vi "Sample Changer 4032 tester.vi"() -> ()   [LabVIEW 2016]
uses:
  Tester-states.ctl
  <vilib>/Utility/file.llb/Write Delimited Spreadsheet (string).vi
  <vilib>/Utility/file.llb/Write Delimited Spreadsheet (I64).vi
  <vilib>/Analysis/NI_AALBase.lvlib
panel:
  in  "file path (dialog if empty)":path
  out "Target Attempts":i32(graph)
  out "Rotation time vs Target Attempts":cluster{i32, i32}[](graph)
  out "Encoder distance":i32
  out "Start Position":i32
  out "output array":cluster{u32, i32}[](array[cluster])
  out "Time vs Distance cluster":cluster{u32, i32}
  out "Rotation time vs Encoder distance":cluster{i32, i32}[](graph)
  in  "Rotation Timeout (ms)":dbl=30000.0
  out "Rotation Duration":u32(graph)
  out "Rotation Duration Histogram":T1(graph)
  out "End Time":timestamp
  out "Start Time":timestamp
  out "Error Histogram":T1(graph)
  out "Success rate":dbl
  out "Sample Number":cluster{"UInt8":u8, "UInt8":u8}(graph)
  in  "Rotate minimum time (ms)":u32=5000
  out "Position error (encoder steps)":i32(graph)
  out "Encoder data":cluster{"Int32":i32, "Int32":i32}(graph)={"Int32"=515, "Int32"=0}
  out "Encoder Destination":i32
  out "Encoder Position":i32
  out "Current Sample":u8
  out "Loop Counter":i32
  in  "Encoder Radius":dbl=2.0
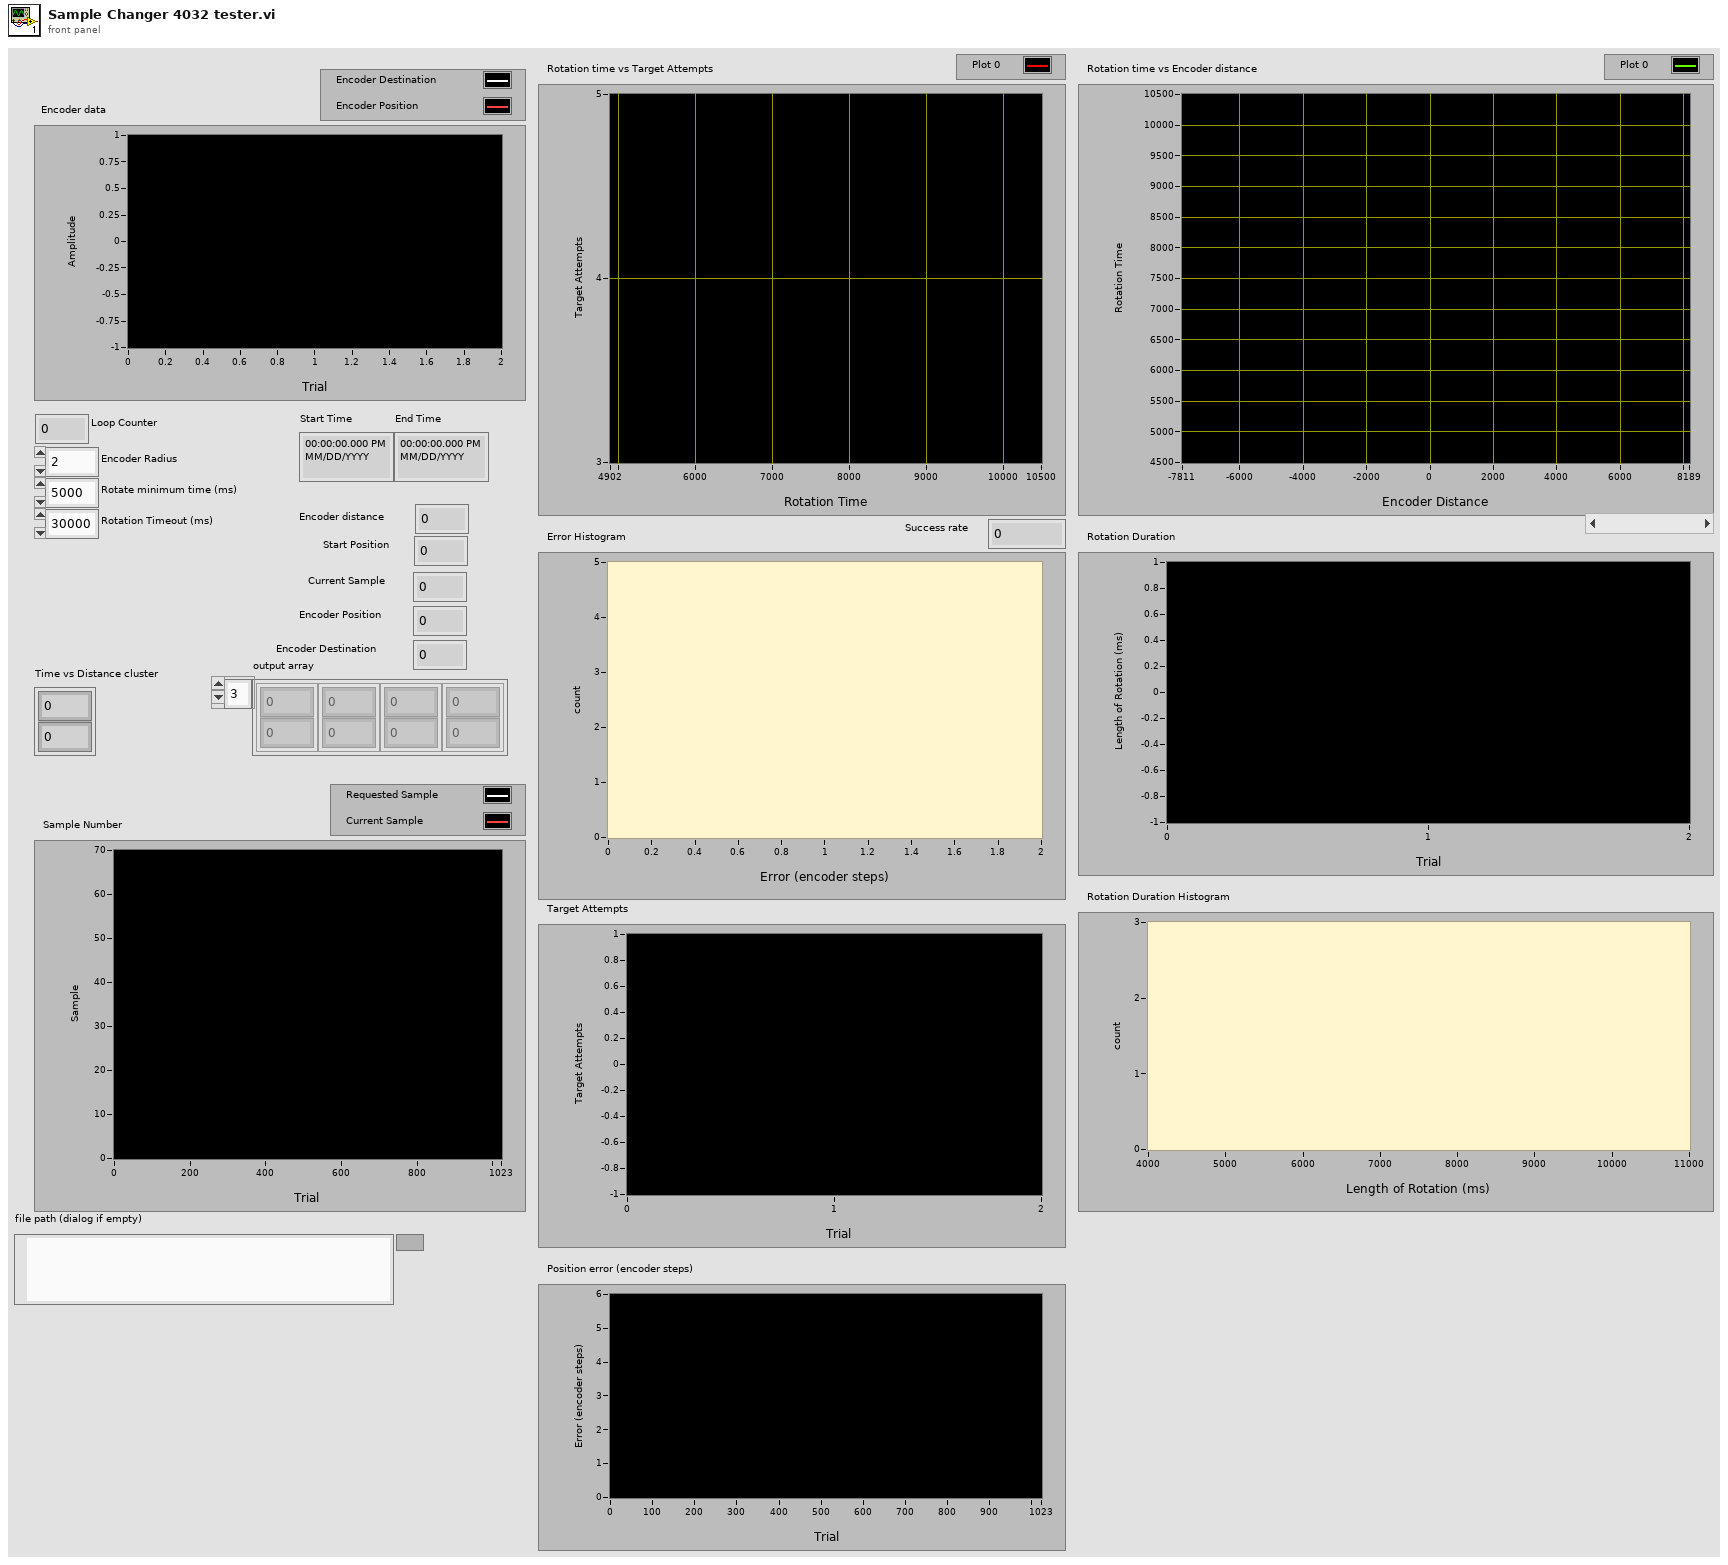
[diagram p1: front panel]
types:
  T1 = cluster{"X Values":dbl[], "Histogram: h(x)":i32[]}
  T2 = typedef "Tester-states.ctl" = enum16{"wait", "start trial", "get trial data", "test complete"}
  T3 = cluster{i32, i32, "Int32":i32, i32, i32, i32, i32}
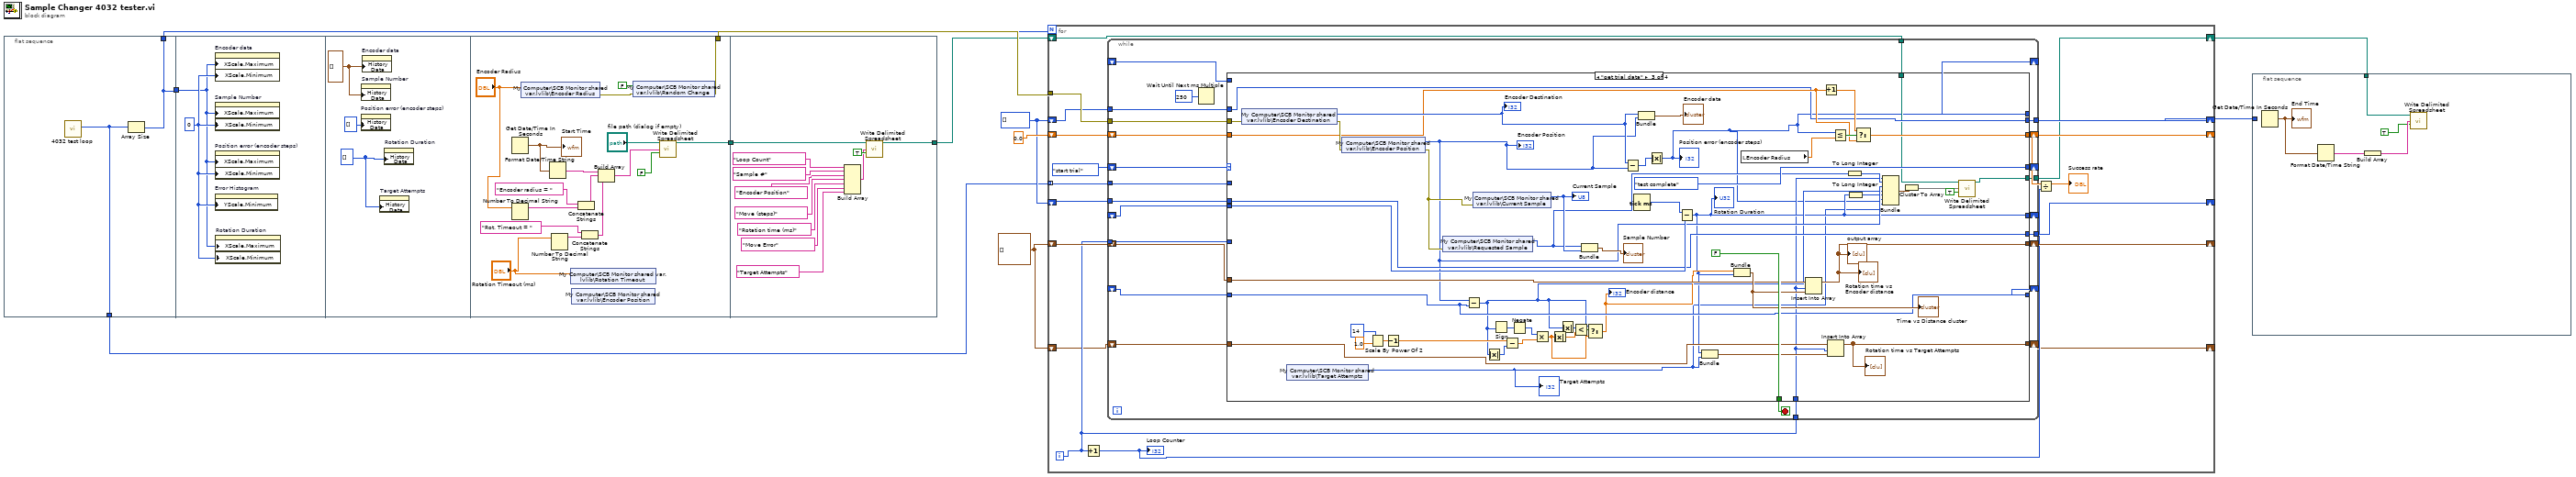
[diagram p0: block diagram]
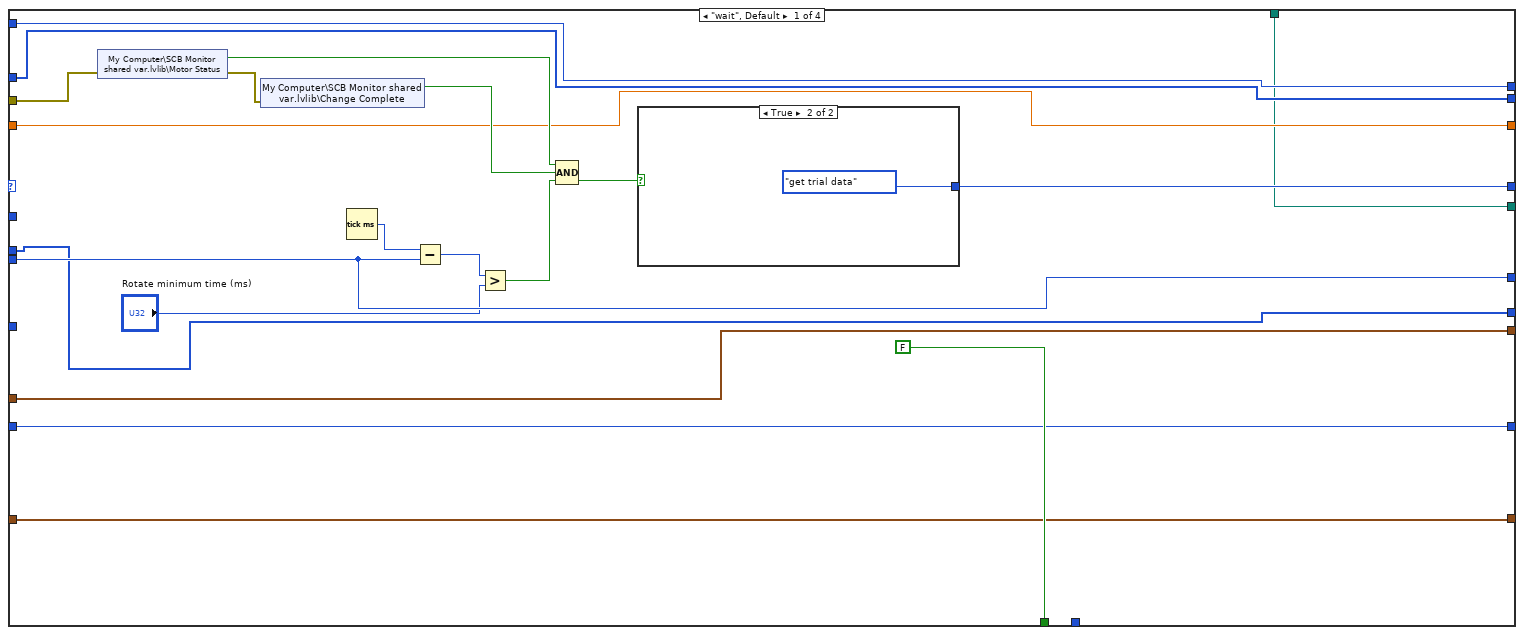
[diagram p2: hidden frame]
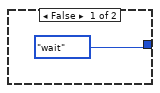
[diagram p3: hidden frame]
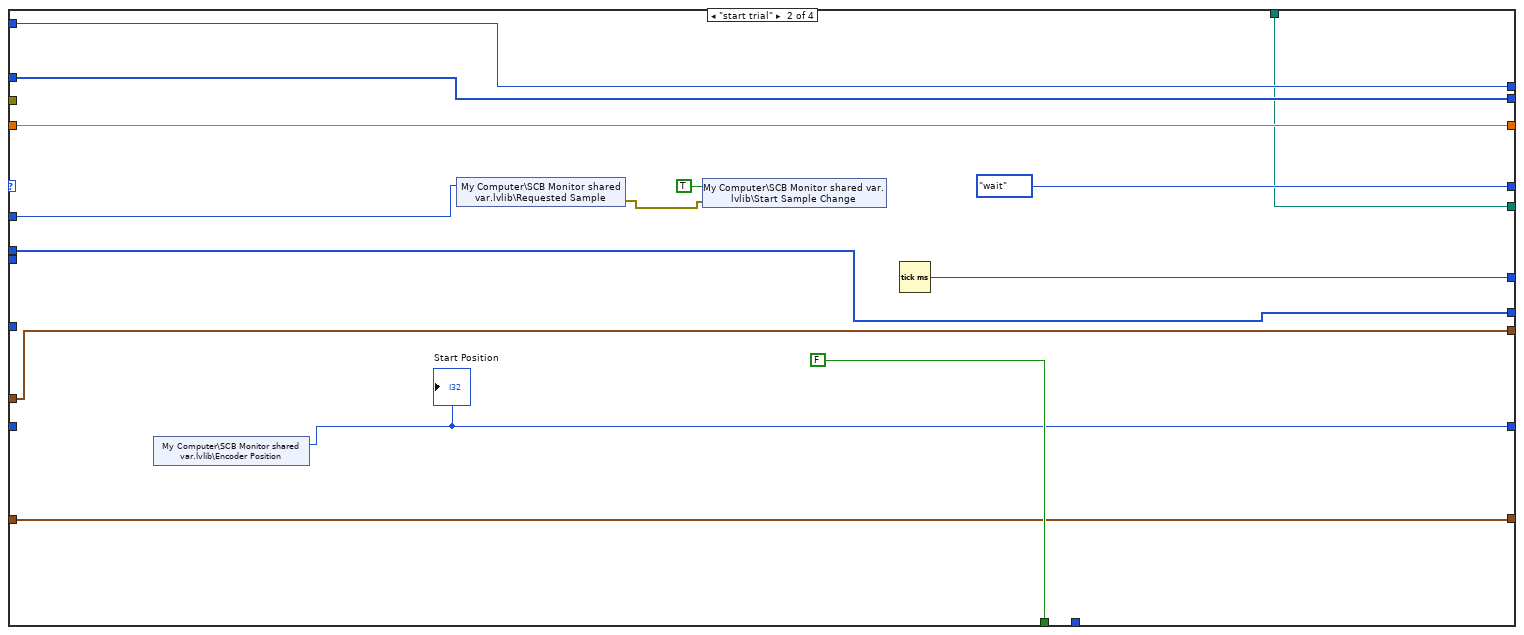
[diagram p4: hidden frame]
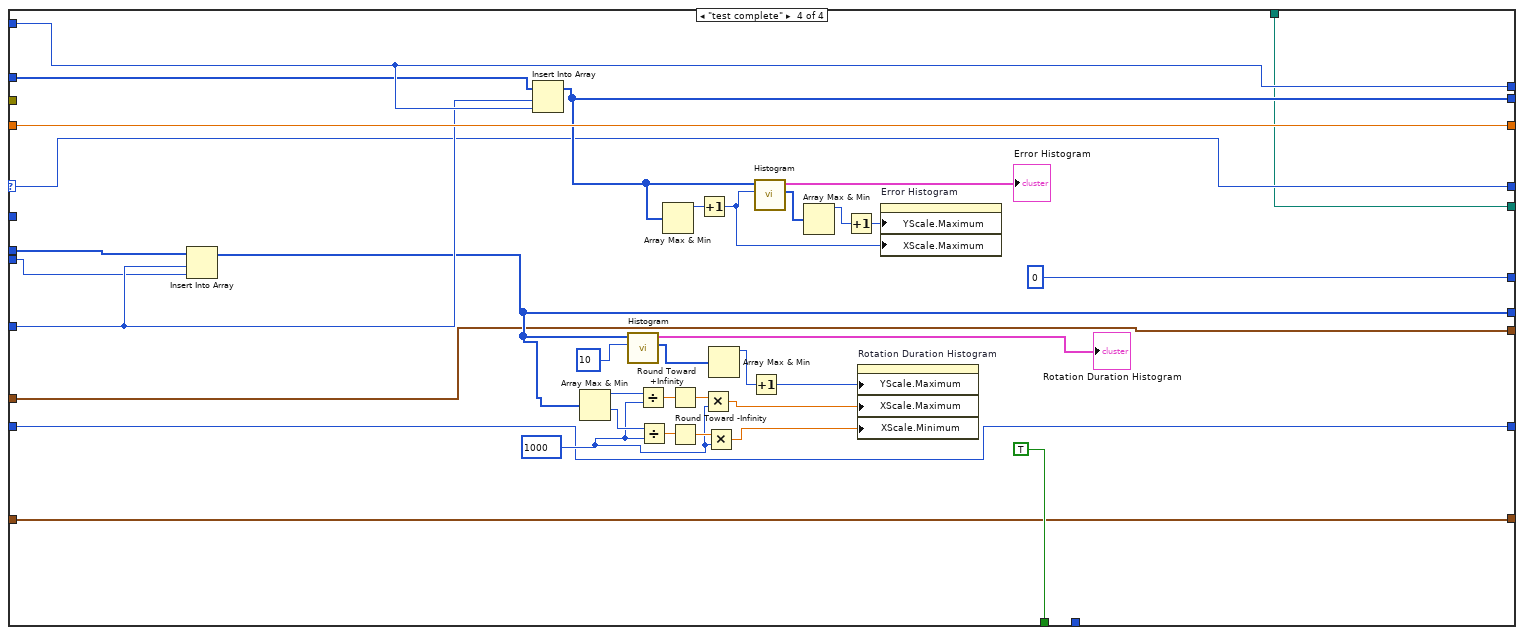
[diagram p5: hidden frame]
diagram:
  w4 = cluster{i32, i32}[] []
  w8 = i32[] []
  n1 = flat-sequence {
    tunnel: [w12] -> w7
    tunnel: [w13] -> w6
    tunnel: [w12] -> w5
    tunnel: w7 -> [w14]
    tunnel: [w33] -> w11
    tunnel: [w31] -> w1
    tunnel: [w45] -> w3
    tunnel: w1 -> [w46]
    frame #0 {
      n2 = call "4032 test loop.vi"() -> ("Array"=w13:i32[])  [unwired: 10 in]
      n3 = Array Size(array=w13) -> (size(s)=w12:i32)
    }
    frame #1 {
      w15 = 0 ("Trials 2")
      n4 = property on="Encoder data" class="WFChart (strict)"("XScale.Maximum"=w14, "XScale.Minimum"=w15) -> ()  [unwired: 2 in, 2 out]
      n5 = property on="Sample Number" class="WFChart (strict)"("XScale.Maximum"=w14, "XScale.Minimum"=w15) -> ()  [unwired: 2 in, 2 out]
      n6 = property on="Position error (encoder steps)" class="WFChart (strict)"("XScale.Maximum"=w14, "XScale.Minimum"=w15) -> ()  [unwired: 2 in, 2 out]
      n7 = property on="Error Histogram" class="XYGraph (strict)"("YScale.Minimum"=w15) -> ()  [unwired: 2 in, 2 out]
      n8 = property on="Rotation Duration" class="WFChart (strict)"("XScale.Maximum"=w14, "XScale.Minimum"=w15) -> ()  [unwired: 2 in, 2 out]
    }
    frame #2 {
      w16 = i32[] [] ("History Data")
      w17 = cluster{"Int32":i32, "Int32":i32}[] [] ("History Data")
      n9 = property on="Position error (encoder steps)" class="WFChart (strict)"("History Data"=i32[] []) -> ()  [unwired: 2 in, 2 out]
      n10 = property on="Sample Number" class="WFChart (strict)"("History Data"=w17) -> ()  [unwired: 2 in, 2 out]
      n11 = property on="Encoder data" class="WFChart (strict)"("History Data"=w17) -> ()  [unwired: 2 in, 2 out]
      n12 = property on="Target Attempts" class="WFChart (strict)"("History Data"=w16) -> ()  [unwired: 2 in, 2 out]
      n13 = property on="Rotation Duration" class="WFChart (strict)"("History Data"=w16) -> ()  [unwired: 2 in, 2 out]
    }
    frame #3 {
      n14 = Get Date/Time In Seconds() -> (seconds since 1Jan1904=w30:timestamp)
      "Start Time" <- w30
      n15 = Number To Decimal String(number="Encoder Radius") -> (decimal integer string=w24:string)  [unwired: 1 in]
      n16 = shared-variable "My Computer\\SCB Monitor shared var.lvlib\\Encoder Radius"("Encoder Radius") -> (error out=w35:errorcluster)  [unwired: 1 in]
      n17 = Format Date/Time String(seconds (now)=w30) -> (date/time string=w29:string)  [unwired: 2 in]
      n18 = Number To Decimal String(number="Rotation Timeout (ms)") -> (decimal integer string=w21:string)  [unwired: 1 in]
      n19 = shared-variable "My Computer\\SCB Monitor shared var.lvlib\\Rotation Timeout"("Rotation Timeout (ms)") -> ()  [unwired: 1 in, 1 out]
      n20 = shared-variable "My Computer\\SCB Monitor shared var.lvlib\\Encoder Position"() -> ()  [unwired: 1 in, 2 out]
      n21 = Concatenate Strings("Encoder radius = ", w24) -> (w23:string)
      n22 = Concatenate Strings("Rot. Timeout = ", w21) -> (w19:string)
      n23 = Build Array(w29, w23, w19) -> (w28:string[])
      n24 = shared-variable "My Computer\\SCB Monitor shared var.lvlib\\Random Change"(FALSE ("Random Change"), error in=w35) -> (error out=w33:errorcluster)
      n25 = call-poly <vilib>:"Write Delimited Spreadsheet.vi"("file path (dialog if empty)"="file path (dialog if empty)", "1D data"=w28, "append to file? (new file:F)"=FALSE) -> ("new file path (Not A Path if cancelled)"=w31:path)  [unwired: 11 in, 1 out]
    }
    frame #4 {
      n26 = Build Array("Loop Count", "Sample #", "Encoder Position", "Move (steps)", "Rotation time (ms)", "Move Error", "Target Attempts" ("element")) -> (w43:string[])
      n27 = call-poly <vilib>:"Write Delimited Spreadsheet.vi"("file path (dialog if empty)"=w46, "1D data"=w43, "append to file? (new file:F)"=TRUE) -> ("new file path (Not A Path if cancelled)"=w45:path)  [unwired: 11 in, 1 out]
    }
  }
  n28 = for {
    N: w5 -> [_]
    tunnel: w11 -> [w63]
    shift-right: [w60] -> _
    shift-left: 0.0 -> [w62]
    shift-right: [w59] -> w9
    shift-left: w8 -> [w58]
    shift-right: [w56] -> _
    shift-left: w8 -> [w57]
    shift-right: [w55] -> _
    shift-left: w4 -> [w54]
    tunnel: w6 -> [w52] mode=indexing
    shift-right: [w49] -> _
    shift-left: w4 -> [w51]
    shift-right: [w47] -> w2
    shift-left: w3 -> [w48]
    i -> [w53]
    n29 = Increment(x=w53) -> (x+1=w50:i32)
    "Loop Counter" <- w50
    n30 = while {
      shift-right: [w88] -> _
      shift-left: Tester-states."start trial" -> [w87]
      tunnel: w63 -> [w86]
      shift-right: [w85] -> _
      shift-left: _ -> [w84]
      shift-right: [w82] -> _
      shift-left: _ -> [w83]
      shift-right: [w81] -> w60
      shift-left: w62 -> [w80]
      tunnel: w53 -> [w79]
      tunnel: [w78] -> w59
      tunnel: w58 -> [w77]
      tunnel: w57 -> [w76]
      tunnel: [w75] -> w56
      tunnel: w53 -> [w71]
      shift-right: [w73] -> w55
      shift-left: w54 -> [w72]
      tunnel: w52 -> [w70]
      shift-right: [w74] -> _
      shift-left: _ -> [w69]
      shift-right: [w68] -> w49
      shift-left: w51 -> [w67]
      tunnel: w48 -> [w66]
      tunnel: [w65] -> w47
      stop <- w90 stop-if-true
      n31 = Wait Until Next ms Multiple(millisecond multiple=u32 250) -> ()  [unwired: 1 out]
      n32 = case shown="\"get trial data\"" w87 {
        selector: w87 -> [_ _ _ w199]
        tunnel: [FALSE FALSE FALSE TRUE] -> w90
        tunnel: [w109 Tester-states."wait" Tester-states."test complete" w199] -> w88
        tunnel: w86 -> [w101 _ w175 _]
        tunnel: [w103 w122 w137 u32 0 ("millisecond timer value")] -> w85
        tunnel: w84 -> [w103 _ w162 w201]
        tunnel: w83 -> [w98 w121 _ w211]
        tunnel: [w98 w121 w127 w211] -> w82
        tunnel: [w97 w120 w167 w212] -> w81
        tunnel: w80 -> [w97 w120 w166 w212]
        tunnel: w79 -> [_ _ _ w202]
        tunnel: [w96 w119 w164 w203] -> w78
        tunnel: w77 -> [w96 w119 w164 w210]
        tunnel: w76 -> [w95 w118 w161 w200]
        tunnel: [w95 w118 w161 w193] -> w75
        tunnel: [w93 w115 w157 w182] -> w74
        tunnel: w69 -> [w93 _ w157 w182]
        tunnel: [w94 w117 w158 w183] -> w73
        tunnel: w72 -> [w94 w117 w159 w183]
        tunnel: w71 -> [_ _ w131 _]
        tunnel: w70 -> [_ w116 _ _]
        tunnel: [w92 w114 w141 w181] -> w68
        tunnel: w67 -> [w92 w114 w142 w181]
        tunnel: w66 -> [w91 w113 w132 w180]
        tunnel: [w91 w113 w130 w180] -> w65
        frame "wait", Default {
          n33 = shared-variable "My Computer\\SCB Monitor shared var.lvlib\\Motor Status"(error in=w101) -> (w102:bool, error out=w100:errorcluster)
          n34 = shared-variable "My Computer\\SCB Monitor shared var.lvlib\\Change Complete"(error in=w100) -> (w106:bool)  [unwired: 1 out]
          n35 = Tick Count (ms)() -> (millisecond timer value=w108:u32)
          n36 = Subtract(x=w108, y=w103) -> (x-y=w105:u32)
          n37 = Greater?(x=w105, y="Rotate minimum time (ms)") -> (0:w104:bool)
          n38 = Compound Arithmetic op=AND(w102, w106, w104) -> (w107:bool)
          n39 = case shown="True" w107 {
            tunnel: [Tester-states."wait" Tester-states."get trial data"] -> w109
            frame False {
            }
            frame True {
            }
          }
        }
        frame "start trial" {
          n40 = shared-variable "My Computer\\SCB Monitor shared var.lvlib\\Encoder Position"() -> (w115:i32)  [unwired: 1 in, 1 out]
          "Start Position" <- w115
          n41 = shared-variable "My Computer\\SCB Monitor shared var.lvlib\\Requested Sample"(w116) -> (error out=w123:errorcluster)  [unwired: 1 in]
          n42 = shared-variable "My Computer\\SCB Monitor shared var.lvlib\\Start Sample Change"(TRUE ("Start Sample Change"), error in=w123) -> ()  [unwired: 1 out]
          n43 = Tick Count (ms)() -> (millisecond timer value=w122:u32)
        }
        frame "get trial data" {
          n44 = shared-variable "My Computer\\SCB Monitor shared var.lvlib\\Encoder Destination"(error in=w175) -> (w173:i32, error out=w174:errorcluster)
          "Encoder Destination" <- w173
          n45 = shared-variable "My Computer\\SCB Monitor shared var.lvlib\\Target Attempts"() -> (w128:i32)  [unwired: 1 in, 1 out]
          "Target Attempts" <- w128
          n46 = shared-variable "My Computer\\SCB Monitor shared var.lvlib\\Encoder Position"(error in=w174) -> (w139:i32, error out=w172:errorcluster)
          "Encoder Position" <- w139
          n47 = Scale By Power Of 2(n=i16 14, x=1.0) -> (x*2^n=w154:dbl)
          n48 = Decrement(x=w154) -> (x-1=w153:dbl)
          n49 = shared-variable "My Computer\\SCB Monitor shared var.lvlib\\Requested Sample"(error in=w172) -> (w140:u8)  [unwired: 1 out]
          n50 = Subtract(x=w139, y=w157) -> (x-y=w138:i32)
          n51 = shared-variable "My Computer\\SCB Monitor shared var.lvlib\\Current Sample"(error in=w172) -> (w170:u8)  [unwired: 1 out]
          "Current Sample" <- w170
          n52 = Absolute Value(x=w138) -> (abs(x)=w152:i32)
          n53 = Sign(1:w138) -> (0:w150:i32)
          n54 = Subtract(x=w153, y=w152) -> (x-y=w151:dbl)
          n55 = Negate(x=w150) -> (-x=w149:i32)
          n56 = Multiply(x=w149, y=w151) -> (x*y=w145:dbl)
          n57 = Absolute Value(x=w145) -> (abs(x)=w148:dbl)
          n58 = Absolute Value(x=w138) -> (abs(x)=w147:i32)
          n59 = Less?(x=w147, y=w148) -> (x < y?=w146:bool)
          n60 = Bundle("UInt8"=w140, "UInt8"=w170) -> (→"Sample Number":cluster{"UInt8":u8, "UInt8":u8})  [unwired: 1 in]
          n61 = Select(t=w138, s=w146, f=w145) -> (s? t:f=w144:dbl)
          "Encoder distance" <- w144
          n62 = Subtract(x=w173, y=w139) -> (x-y=w177:i32)
          n63 = Tick Count (ms)() -> (millisecond timer value=w163:u32)
          n64 = Bundle("Int32"=w173, "Int32"=w139) -> (→"Encoder data":cluster{"Int32":i32, "Int32":i32})  [unwired: 1 in]
          n65 = Absolute Value(x=w177) -> (abs(x)=w127:i32)
          "Position error (encoder steps)" <- w127
          n66 = Subtract(x=w163, y=w162) -> (x-y=w137:u32)
          "Rotation Duration" <- w137
          n67 = Bundle(w137, w128) -> (w143:cluster{u32, i32})  [unwired: 1 in]
          n68 = Bundle(w144, w137) -> (w160:cluster{dbl, u32})  [unwired: 1 in]
          "Time vs Distance cluster" <- w160
          n69 = local read "Encoder Radius"() -> (w169:dbl)
          n70 = Insert Into Array(array=w159, index=w131, new element=w160) -> (w158:cluster{i32, i32}[])
          "Rotation time vs Encoder distance" <- w158
          "output array" <- w158
          n71 = Increment(x=w166) -> (x+1=w165:dbl)
          n72 = Insert Into Array(array=w142, index=w131, new element=w143) -> (w141:cluster{i32, i32}[])
          "Rotation time vs Target Attempts" <- w141
          n73 = Less Or Equal?(x=w127, y=w169) -> (x <= y?=w168:bool)
          n74 = To Long Integer(number=w140) -> (32bit integer=w136:i32)
          n75 = To Long Integer(number=w137) -> (32bit integer=w135:i32)
          n76 = Select(t=w165, s=w168, f=w166) -> (s? t:f=w167:dbl)
          n77 = Bundle(w131, w136, "Int32"=w139, w138, w135, w127, w128) -> (w134:T3)  [unwired: 1 in]
          n78 = Cluster To Array(cluster=w134) -> (array=w133:i32[])
          n79 = call-poly <vilib>:"Write Delimited Spreadsheet.vi"("file path (dialog if empty)"=w132, "1D data"=w133, "append to file? (new file:F)"=TRUE) -> ("new file path (Not A Path if cancelled)"=w130:path)  [unwired: 11 in, 1 out]
        }
        frame "test complete" {
          w186 = 1000 ("y")
          n80 = Insert Into Array(array=w200, index=w202, new element=w201) -> (w193:i32[])
          n81 = Insert Into Array(array=w210, index=w202, new element=w211) -> (w203:i32[])
          n82 = Array Max & Min(array=w193) -> (max value=w192:i32, min value=w191:i32)  [unwired: 2 out]
          n83 = call <vilib>:"Histogram.vi"("intervals"=10, "X"=w193) -> ("Histogram: h(x)"=w195:i32[], "Histogram Graph"=→"Rotation Duration Histogram":T1)  [unwired: 6 in, 2 out]
          n84 = Divide(x=w192, y=w186) -> (x/y=w189:dbl)
          n85 = Divide(x=w191, y=w186) -> (x/y=w190:dbl)
          n86 = Array Max & Min(array=w203) -> (max value=w209:i32)  [unwired: 3 out]
          n87 = Round Toward +Infinity(x=w189) -> (ceil(x): smallest int >= x=w188:dbl)
          n88 = Round Toward -Infinity(1:w190) -> (0:w187:dbl)
          n89 = Increment(x=w209) -> (x+1=w204:i32)
          n90 = Multiply(x=w188, y=w186) -> (x*y=w185:dbl)
          n91 = Multiply(x=w187, y=w186) -> (x*y=w184:dbl)
          n92 = Array Max & Min(array=w195) -> (max value=w196:i32)  [unwired: 3 out]
          n93 = Increment(x=w196) -> (x+1=w194:i32)
          n94 = call <vilib>:"Histogram.vi"("intervals"=w204, "X"=w203) -> ("Histogram: h(x)"=w207:i32[], "Histogram Graph"=→"Error Histogram":T1)  [unwired: 6 in, 2 out]
          n95 = Array Max & Min(array=w207) -> (max value=w206:i32)  [unwired: 3 out]
          n96 = Increment(x=w206) -> (x+1=w205:i32)
          n97 = property on="Rotation Duration Histogram" class="XYGraph (strict)"("YScale.Maximum"=w194, "XScale.Maximum"=w185, "XScale.Minimum"=w184) -> ()  [unwired: 2 in, 2 out]
          n98 = property on="Error Histogram" class="XYGraph (strict)"("YScale.Maximum"=w205, "XScale.Maximum"=w204) -> ()  [unwired: 2 in, 2 out]
        }
      }
    }
    n99 = Divide(x=w60, y=w50) -> (x/y=→"Success rate":dbl)
  }
  n100 = flat-sequence {
    tunnel: w9 -> [_]
    tunnel: w2 -> [w215]
    frame #0 {
      n101 = Get Date/Time In Seconds() -> (seconds since 1Jan1904=w218:timestamp)
      "End Time" <- w218
      n102 = Format Date/Time String(seconds (now)=w218) -> (date/time string=w219:string)  [unwired: 2 in]
      n103 = Build Array(w219) -> (w217:string[])
      n104 = call-poly <vilib>:"Write Delimited Spreadsheet.vi"("file path (dialog if empty)"=w215, "1D data"=w217, "append to file? (new file:F)"=TRUE) -> ()  [unwired: 11 in, 2 out]
    }
  }
